vi "_decrementHeadIndex.vi"(11 "VariantBuffer in":refnum<class "VariantBuffer.lvclass">) -> (3 "VariantBuffer out":refnum<class "VariantBuffer.lvclass">)   [LabVIEW 2013, in "CircularBuffer.lvlib" / "VariantBuffer.lvclass"]
uses:
  VariantBuffer.lvclass
  VariantBuffer.lvclass/VariantBuffer.ctl
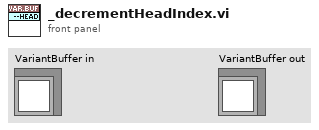
[diagram p1: front panel]
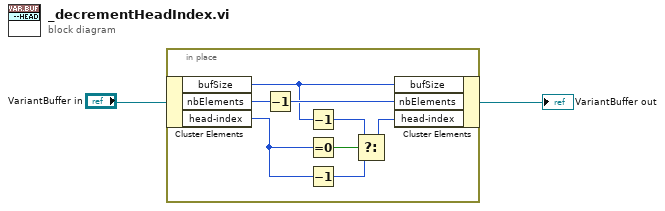
[diagram p0: block diagram]
diagram:
  n1 = in-place {
    n2 = in-place-cluster #1("VariantBuffer in") -> ("bufSize"=w4:i32, "nbElements"=w10:i32, "head-index"=w5:i32)
    n3 = Decrement(x=w10) -> (x-1=w9:i32)
    n4 = Decrement(x=w4) -> (x-1=w6:i32)
    n5 = Equal To 0?(x=w5) -> (x = 0?=w7:bool)
    n6 = Decrement(x=w5) -> (x-1=w8:i32)
    n7 = Select(t=w6, s=w7, f=w8) -> (s? t:f=w3:i32)
    n8 = in-place-cluster #1("bufSize"=w4, "nbElements"=w9, "head-index"=w3) -> (→"VariantBuffer out":refnum<class "VariantBuffer.lvclass">)
  }
